vi "ClientLog.vi"(8 "error in (no error)":errorcluster, 10 "User and Project Inputs":T3, 11 "DesignRequest":T2) -> (0 "error out":errorcluster)   [LabVIEW 2011]
uses:
  Variable cluster.ctl
  Design Request.ctl
  RequestKeys.ctl
  Design Server.lvlib
panel:
  in  "Request Keys":T1=enum."ProjectNotes"
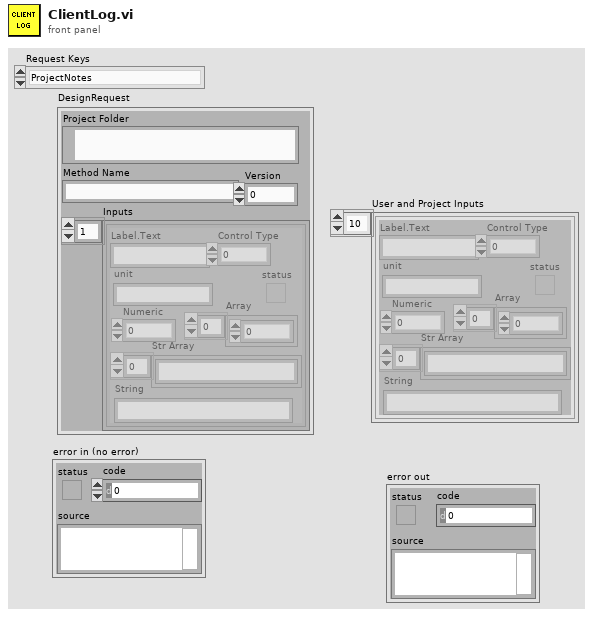
[diagram p1: front panel]
types:
  T1 = typedef "Design Server.lvlib/RequestKeys.ctl" = enum16{"FormName", "Name", "Email", "Organization", "Country", "ProjectTitle", "ProjectCity", "ProjectState", "ProjectNotes"}
  T2 = typedef "Design Server.lvlib/Design Request.ctl" = cluster{"Project Folder":path, "Method Name":string, "Inputs":T3, "Version":i32}
  T3 = typedef "Design Server.lvlib/Variable cluster.ctl" = cluster{"Label.Text":string, "Control Type":u32, "Numeric":dbl, "Array":dbl[], "status":bool, "Str Array":string[], "String":string, "unit":string}[]
  T4 = enum16{"open", "replace", "create", "open or create", "replace or create", "replace or create with confirmation"}
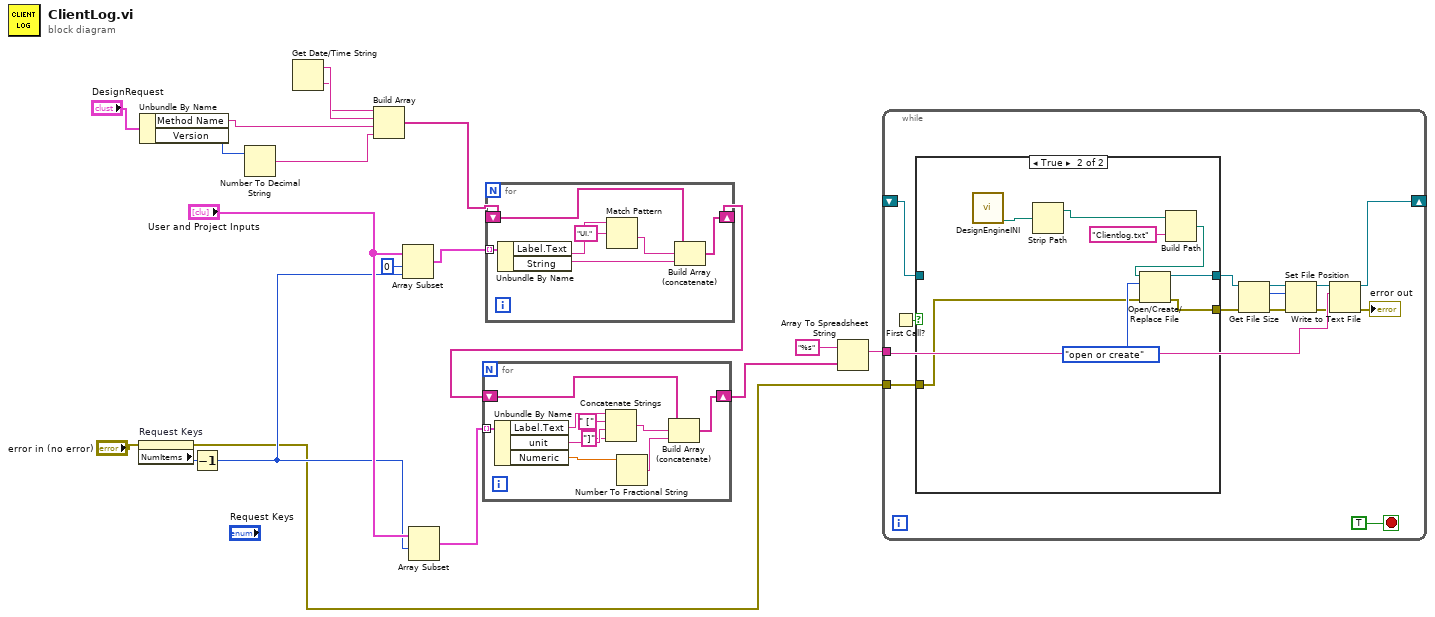
[diagram p0: block diagram]
diagram:
  n1 = property on="Request Keys" class="Enum (strict)"(error in="error in (no error)") -> (error out=w3:errorcluster, "NumItems"=w17:u32)  [unwired: 1 in, 1 out]
  n2 = Unbundle By Name("DesignRequest") -> ("Method Name"=w9:string, "Version"=w18:i32)
  n3 = Decrement(x=w17) -> (x-1=w12:u32)
  n4 = Number To Decimal String(number=w18) -> (decimal integer string=w8:string)  [unwired: 1 in]
  n5 = Get Date/Time String() -> (date string=w2:string, time string=w1:string)  [unwired: 3 in]
  n6 = Build Array(w1, w2, w9, w8) -> (w6:string[])
  n7 = Array Subset(array="User and Project Inputs", index=0, length=w12) -> (w13:T3)
  n8 = Array Subset(array="User and Project Inputs", index=w12) -> (w16:T3)  [unwired: 1 in]
  n9 = for {
    tunnel: w13 -> [w26] mode=indexing
    shift-right: [w25] -> w10
    shift-left: w6 -> [w24]
    n10 = Unbundle By Name(w26) -> ("Label.Text"=w22:string, "String"=w23:string)
    n11 = Match Pattern(string=w22, regular expression="UI.") -> (after substring=w20:string)  [unwired: 1 in, 3 out]
    n12 = Build Array (concatenate)(w24, w20, w23) -> (w25:string[])
  }
  n13 = for {
    tunnel: w16 -> [w36] mode=indexing
    shift-right: [w33] -> w5
    shift-left: w10 -> [w32]
    n14 = Unbundle By Name(w36) -> ("Label.Text"=w31:string, "unit"=w29:string, "Numeric"=w35:dbl)
    n15 = Concatenate Strings(w31, " [" ("string"), w29, "]" ("string")) -> (w27:string)
    n16 = Number To Fractional String(number=w35) -> (F-format string=w34:string)  [unwired: 3 in]
    n17 = Build Array (concatenate)(w32, w27, w34) -> (w33:string[])
  }
  n18 = Array To Spreadsheet String(array=w5, 3:"%s" ("format string")) -> (spreadsheet string=w15:string)  [unwired: 1 in]
  n19 = while {
    tunnel: w15 -> [w50]
    shift-right: [w42] -> _
    shift-left: _ -> [w40]
    tunnel: w3 -> [w37]
    stop <- TRUE stop-if-true
    n20 = First Call?() -> (First Call?: T/F=w44:bool)
    n21 = case shown="True" w44 {
      tunnel: [w52 w57] -> w43
      tunnel: [w51 w56] -> w41
      tunnel: w40 -> [w52 _]
      tunnel: w37 -> [w51 w55]
      frame False {
      }
      frame True {
        n22 = call "DesignEngineINI.vi"() -> ("Ini file path"=w54:path)  [unwired: 6 in, 1 out]
        n23 = Strip Path(path=w54) -> (stripped path=w53:path)  [unwired: 1 out]
        n24 = Build Path(base path=w53, name or relative path="Clientlog.txt") -> (appended path=w58:path)
        n25 = Open/Create/Replace File(file path (use dialog)=w58, error in=w55, operation (0:open)=T4."open or create") -> (refnum out=w57:refnum<file>, error out=w56:errorcluster)  [unwired: 3 in, 1 out]
      }
    }
    n26 = Get File Size(file=w43, error in=w41) -> (refnum out=w49:refnum<file>, size (in bytes)=w45:i64, 0:w48:errorcluster)
    n27 = Set File Position(offset (in bytes) (0)=w45, refnum=w49, error in=w48) -> (refnum out=w47:refnum<file>, error out=w46:errorcluster)  [unwired: 1 in]
    n28 = Write to Text File(file (use dialog)=w47, text=w50, error in=w46) -> (refnum out=w42:refnum<file>, error out=→"error out":errorcluster)  [unwired: 1 in, 1 out]
  }
